vi "notes.add.vi"(8 "error in (no error)":errorcluster, 10 "midi-file-events":refnum<class "midi-file-events.lvclass">, 11 "midi-ui in":refnum<class "midi-ui.lvclass">) -> (0 "error out":errorcluster, 3 "midi-ui out":refnum<class "midi-ui.lvclass">)   [LabVIEW 2020, in "midi-ui.lvclass"]
uses:
  midi-ui.lvclass
  midi-file-events/midi-file-events.lvclass
  midi-ui.lvclass/midi-ui.ctl
  midi-file-event.midi/midi-file-event.midi.lvclass/midi-file-event.midi.ctl
  midi-file-event/midi-file-event.lvclass/midi-file-event.ctl
  midi-file-event.midi/MIDI_Messages.get.vi
  midi-file-event.midi/Data1.get.vi
  midi-file-event.midi/Data2.get.vi
  midi-file-event/uid.get.vi
  midi-file-event.midi/midi-file-event.midi.lvclass
  C:/code/LabVIEW-MIDI/lv-src/midi-file-event/midi-file-event.lvclass
  shared/midi note number.ctl
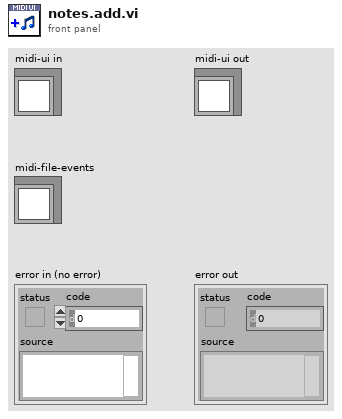
[diagram p1: front panel]
types:
  T1 = map{i32, cluster{"Note On":picture, "Note Off":picture}}
  T2 = typedef "midi-ui.lvclass/privatedata.ctl" = cluster{"White Key Length":dbl, "White Key Width":dbl, "Black Key Length":dbl, "Key Polygon Corners by Name":map{string, cluster{"x":dbl, "y":dbl}[]}, "Anticlockwise rotations [0-3] (0)":i32, "Polygon Corners by Note Name":map{T3, cluster{"x":dbl, "y":dbl}[]}, "Picture Control":refnum<vi>, "Owning VI":refnum<vi>, "Control Index":i32, "Keyboard Key Note Bounds by Note Name":map{T3, cluster{"max":dbl, "min":dbl}}, "Notes on screen":cluster{"Note":T3, "End Time":u32, "Start Time":u32}[], "Polygon Pictures by Note Name":map{T3, cluster{"Note On":picture, "Note Off":picture}}, "keyboard":picture[], "Keyboard Note Picture Index by Name":map{T3, i32}, "music":picture[], "Zoom Factor":sgl}
  T3 = typedef "midi note number.ctl" = enum8{"0 - C-1 - 8.18", "1 - C#-1 - 8.66", "2 - D-1 - 9.18", "3 - D#-1 - 9.72", "4 - E-1 - 10.30", "5 - F-1 - 10.91", "6 - F#-1 - 11.56", "7 - G-1 - 12.25", "8 - G#-1 - 12.98", "9 - A-1 - 13.75", "10 - A#-1 - 14.57", "11 - B-1 - 15.43", "12 - C0 - 16.35", "13 - C#0 - 17.32", "14 - D0 - 18.35", "15 - D#0 - 19.45", "16 - E0 - 20.60", "17 - F0 - 21.83", "18 - F#0 - 23.12", "19 - G0 - 24.50", "20 - G#0 - 25.96", "21 - A0 - 27.50", "22 - A#0 - 29.14", "23 - B0 - 30.87", "24 - C1 - 32.70", "25 - C#1 - 34.65", "26 - D1 - 36.71", "27 - D#1 - 38.89", "28 - E1 - 41.20", "29 - F1 - 43.65", "30 - F#1 - 46.25", "31 - G1 - 49.00", "32 - G#1 - 51.91", "33 - A1 - 55.00", "34 - A#1 - 58.27", "35 - B1 - 61.74", "36 - C2 - 65.41", "37 - C#2 - 69.30", "38 - D2 - 73.42", "39 - D#2 - 77.78", "40 - E2 - 82.41", "41 - F2 - 87.31", "42 - F#2 - 92.50", "43 - G2 - 98.00", "44 - G#2 - 103.83", "45 - A2 - 110.00", "46 - A#2 - 116.54", "47 - B2 - 123.47", "48 - C3 - 130.81", "49 - C#3 - 138.59", "50 - D3 - 146.83", "51 - D#3 - 155.56", "52 - E3 - 164.81", "53 - F3 - 174.61", "54 - F#3 - 185.00", "55 - G3 - 196.00", "56 - G#3 - 207.65", "57 - A3 - 220.00", "58 - A#3 - 233.08", "59 - B3 - 246.94", "60 - C4 - 261.63", "61 - C#4 - 277.18", "62 - D4 - 293.66", "63 - D#4 - 311.13", "64 - E4 - 329.63", "65 - F4 - 349.23", "66 - F#4 - 369.99", "67 - G4 - 392.00", "68 - G#4 - 415.30", "69 - A4 - 440.00", "70 - A#4 - 466.16", "71 - B4 - 493.88", "72 - C5 - 523.25", "73 - C#5 - 554.37", "74 - D5 - 587.33", "75 - D#5 - 622.25", "76 - E5 - 659.25", "77 - F5 - 698.46", "78 - F#5 - 739.99", "79 - G5 - 783.99", "80 - G#5 - 830.61", "81 - A5 - 880.00", "82 - A#5 - 932.33", "83 - B5 - 987.77", "84 - C6 - 1046.50", "85 - C#6 - 1108.73", "86 - D6 - 1174.66", "87 - D#6 - 1244.51", "88 - E6 - 1318.51", "89 - F6 - 1396.91", "90 - F#6 - 1479.98", "91 - G6 - 1567.98", "92 - G#6 - 1661.22", "93 - A6 - 1760.00", "94 - A#6 - 1864.66", "95 - B6 - 1975.53", "96 - C7 - 2093.00", "97 - C#7 - 2217.46", "98 - D7 - 2349.32", "99 - D#7 - 2489.02", "100 - E7 - 2637.02", "101 - F7 - 2793.83", "102 - F#7 - 2959.96", "103 - G7 - 3135.96", "104 - G#7 - 3322.44", "105 - A7 - 3520.00", "106 - A#7 - 3729.31", "107 - B7 - 3951.07", "108 - C8 - 4186.01", "109 - C#8 - 4434.92", "110 - D8 - 4698.63", "111 - D#8 - 4978.03", "112 - E8 - 5274.04", "113 - F8 - 5587.65", "114 - F#8 - 5919.91", "115 - G8 - 6271.93", "116 - G#8 - 6644.88", "117 - A8 - 7040.00", "118 - A#8 - 7458.62", "119 - B8 - 7902.13", "120 - C9 - 8372.02", "121 - C#9 - 8869.84", "122 - D9 - 9397.27", "123 - D#9 - 9956.06", "124 - E9 - 10548.08", "125 - F9 - 11175.30", "126 - F#9 - 11839.82", "127 - G9 - 12543.85"}
  T4 = cluster{"left":i16, "top":i16, "right":i16, "bottom":i16}
  T5 = cluster{"Note":T3, "End Time":u32, "Start Time":u32, "on uid":string, "off uid":string}
  T6 = map{T3, cluster{"Note":T3, "End Time":u32, "Start Time":u32, "on uid":string, "off uid":string}}
  T7 = map{dbl, set{refnum<class "midi-file-event.midi.lvclass">}}
  T8 = set{refnum<class "midi-file-event.midi.lvclass">}
  T9 = typedef "midi-file.lvclass/MIDI Messages.ctl" = enum8{"0(0x00)_UnassignedMidiMessage", "1(0x01)_UnassignedMidiMessage", "2(0x02)_UnassignedMidiMessage", "3(0x03)_UnassignedMidiMessage", "4(0x04)_UnassignedMidiMessage", "5(0x05)_UnassignedMidiMessage", "6(0x06)_UnassignedMidiMessage", "7(0x07)_UnassignedMidiMessage", "8(0x08)_NoteOffEvent", "9(0x09)_NoteOnEvent", "10(0x0A)_PolyphonicKeyPressure", "11(0x0B)_ControlChange", "12(0x0C)_ProgramChange", "13(0x0D)_ChannelPressure", "14(0x0E)_PitchBendChange", "15(0x0F)_SystemExclusive(SysEx)", "16(0x10)_UnassignedMidiMessage", "17(0x11)_UnassignedMidiMessage", "18(0x12)_UnassignedMidiMessage", "19(0x13)_UnassignedMidiMessage", "20(0x14)_UnassignedMidiMessage", "21(0x15)_UnassignedMidiMessage", "22(0x16)_UnassignedMidiMessage", "23(0x17)_UnassignedMidiMessage", "24(0x18)_UnassignedMidiMessage", "25(0x19)_UnassignedMidiMessage", "26(0x1A)_UnassignedMidiMessage", "27(0x1B)_UnassignedMidiMessage", "28(0x1C)_UnassignedMidiMessage", "29(0x1D)_UnassignedMidiMessage", "30(0x1E)_UnassignedMidiMessage", "31(0x1F)_UnassignedMidiMessage", "32(0x20)_UnassignedMidiMessage", "33(0x21)_UnassignedMidiMessage", "34(0x22)_UnassignedMidiMessage", "35(0x23)_UnassignedMidiMessage", "36(0x24)_UnassignedMidiMessage", "37(0x25)_UnassignedMidiMessage", "38(0x26)_UnassignedMidiMessage", "39(0x27)_UnassignedMidiMessage", "40(0x28)_UnassignedMidiMessage", "41(0x29)_UnassignedMidiMessage", "42(0x2A)_UnassignedMidiMessage", "43(0x2B)_UnassignedMidiMessage", "44(0x2C)_UnassignedMidiMessage", "45(0x2D)_UnassignedMidiMessage", "46(0x2E)_UnassignedMidiMessage", "47(0x2F)_UnassignedMidiMessage", "48(0x30)_UnassignedMidiMessage", "49(0x31)_UnassignedMidiMessage", "50(0x32)_UnassignedMidiMessage", "51(0x33)_UnassignedMidiMessage", "52(0x34)_UnassignedMidiMessage", "53(0x35)_UnassignedMidiMessage", "54(0x36)_UnassignedMidiMessage", "55(0x37)_UnassignedMidiMessage", "56(0x38)_UnassignedMidiMessage", "57(0x39)_UnassignedMidiMessage", "58(0x3A)_UnassignedMidiMessage", "59(0x3B)_UnassignedMidiMessage", "60(0x3C)_UnassignedMidiMessage", "61(0x3D)_UnassignedMidiMessage", "62(0x3E)_UnassignedMidiMessage", "63(0x3F)_UnassignedMidiMessage", "64(0x40)_UnassignedMidiMessage", "65(0x41)_UnassignedMidiMessage", "66(0x42)_UnassignedMidiMessage", "67(0x43)_UnassignedMidiMessage", "68(0x44)_UnassignedMidiMessage", "69(0x45)_UnassignedMidiMessage", "70(0x46)_UnassignedMidiMessage", "71(0x47)_UnassignedMidiMessage", "72(0x48)_UnassignedMidiMessage", "73(0x49)_UnassignedMidiMessage", "74(0x4A)_UnassignedMidiMessage", "75(0x4B)_UnassignedMidiMessage", "76(0x4C)_UnassignedMidiMessage", "77(0x4D)_UnassignedMidiMessage", "78(0x4E)_UnassignedMidiMessage", "79(0x4F)_UnassignedMidiMessage", "80(0x50)_UnassignedMidiMessage", "81(0x51)_UnassignedMidiMessage", "82(0x52)_UnassignedMidiMessage", "83(0x53)_UnassignedMidiMessage", "84(0x54)_UnassignedMidiMessage", "85(0x55)_UnassignedMidiMessage", "86(0x56)_UnassignedMidiMessage", "87(0x57)_UnassignedMidiMessage", "88(0x58)_UnassignedMidiMessage", "89(0x59)_UnassignedMidiMessage", "90(0x5A)_UnassignedMidiMessage", "91(0x5B)_UnassignedMidiMessage", "92(0x5C)_UnassignedMidiMessage", "93(0x5D)_UnassignedMidiMessage", "94(0x5E)_UnassignedMidiMessage", "95(0x5F)_UnassignedMidiMessage", "96(0x60)_UnassignedMidiMessage", "97(0x61)_UnassignedMidiMessage", "98(0x62)_UnassignedMidiMessage", "99(0x63)_UnassignedMidiMessage", "100(0x64)_UnassignedMidiMessage", "101(0x65)_UnassignedMidiMessage", "102(0x66)_UnassignedMidiMessage", "103(0x67)_UnassignedMidiMessage", "104(0x68)_UnassignedMidiMessage", "105(0x69)_UnassignedMidiMessage", "106(0x6A)_UnassignedMidiMessage", "107(0x6B)_UnassignedMidiMessage", "108(0x6C)_UnassignedMidiMessage", "109(0x6D)_UnassignedMidiMessage", "110(0x6E)_UnassignedMidiMessage", "111(0x6F)_UnassignedMidiMessage", "112(0x70)_UnassignedMidiMessage", "113(0x71)_UnassignedMidiMessage", "114(0x72)_UnassignedMidiMessage", "115(0x73)_UnassignedMidiMessage", "116(0x74)_UnassignedMidiMessage", "117(0x75)_UnassignedMidiMessage", "118(0x76)_UnassignedMidiMessage", "119(0x77)_UnassignedMidiMessage", "120(0x78)_UnassignedMidiMessage", "121(0x79)_UnassignedMidiMessage", "122(0x7A)_UnassignedMidiMessage", "123(0x7B)_UnassignedMidiMessage", "124(0x7C)_UnassignedMidiMessage", "125(0x7D)_UnassignedMidiMessage", "126(0x7E)_UnassignedMidiMessage", "127(0x7F)_UnassignedMidiMessage"}
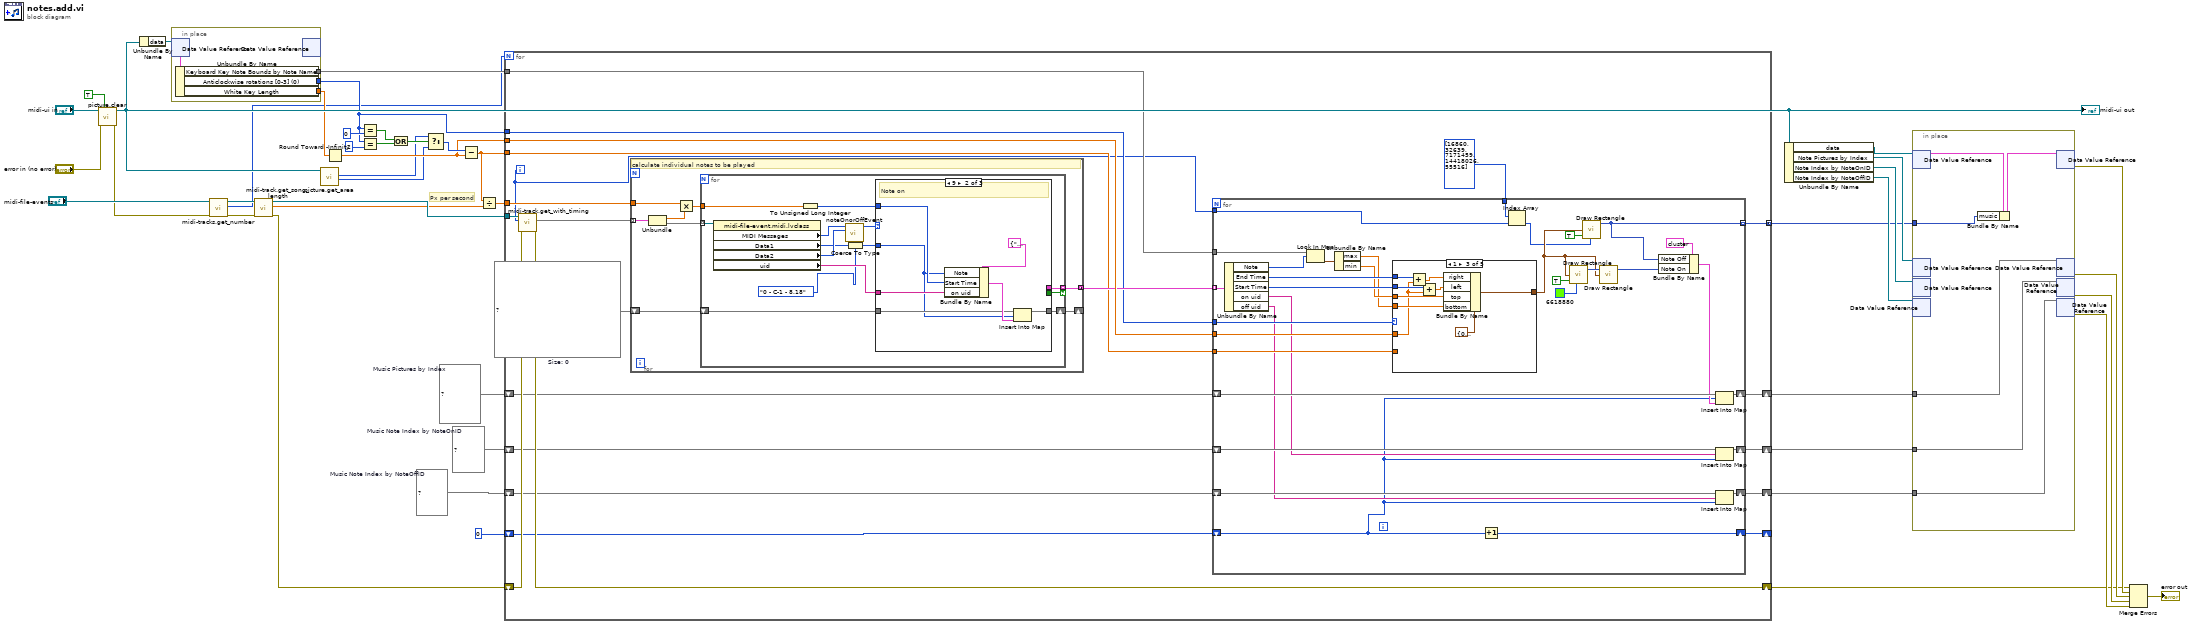
[diagram p0: block diagram]
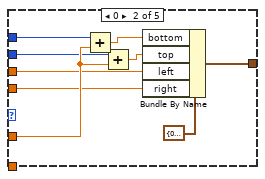
[diagram p3: hidden frame]
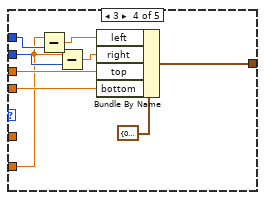
[diagram p4: hidden frame]
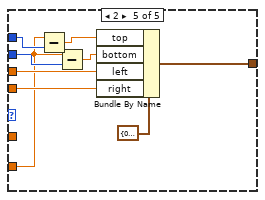
[diagram p5: hidden frame]
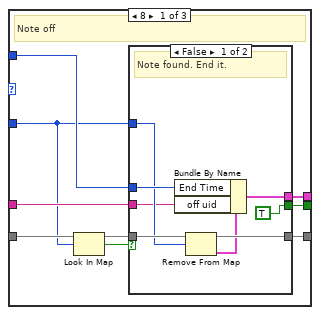
[diagram p6: hidden frame]
diagram:
  w7 = map{string, i32} {}  # Music Note Index by NoteOffID
  w9 = T1 {}  # Music Pictures by Index
  w8 = map{string, i32} {}  # Music Note Index by NoteOnID
  # "Px per second"
  n1 = call "picture.clear.vi"("Keep Keyboard? (T)"=TRUE, "error in"="error in (no error)", "midi-ui in"="midi-ui in") -> ("error out"=w14:errorcluster, "midi-ui out"=w32:refnum<class "midi-ui.lvclass">)  [unwired: 7 in]
  "midi-ui out" <- w32
  n2 = Unbundle By Name(w32) -> ("data"=w31:refnum<data-value>)
  n3 = in-place {
    in-place-border: [w48] -> w30
    in-place-border: [w47] -> w29
    in-place-border: [w46] -> w28
    n4 = in-place-dvr #1(w31) -> (w49:T2)  [unwired: 1 out]
    n5 = Unbundle By Name(w49) -> ("Keyboard Key Note Bounds by Note Name"=w46:map{T3, cluster{"max":dbl, "min":dbl}}, "Anticlockwise rotations [0-3] (0)"=w48:i32, "White Key Length"=w47:dbl)
    n6 = in-place-dvr #1() -> ()  [unwired: 1 in, 2 out]
  }
  n7 = call "midi-tracks.get_number.vi"("error in (no error)"=w14, "midi-file-events in"="midi-file-events") -> ("error out"=w17:errorcluster, "Numer of Tracks"=w10:i32, "midi-file-events out"=w18:refnum<class "midi-file-events.lvclass">)  [unwired: 7 in]
  n8 = call "midi-track.get_song_length.vi"("error in (no error)"=w17, "midi-file-events in"=w18) -> ("error out"=w16:errorcluster, "Song Length (s)"=w11:dbl, "midi-file-events out"=w15:refnum<class "midi-file-events.lvclass">)  [unwired: 7 in]
  n9 = call "picture.get_area.vi"("midi-ui in"=w32) -> ("Bounds:Area Width"=w33:u32, "Bounds:Area Height"=w34:u32)  [unwired: 7 in, 2 out]
  n10 = Round Toward -Infinity(1:w29) -> (0:w38:dbl)
  n11 = Equal?(x=w30, y=0) -> (x = y?=w43:bool)
  n12 = Equal?(x=w30, y=2) -> (x = y?=w42:bool)
  n13 = Or(x=w43, y=w42) -> (x .or. y?=w41:bool)
  n14 = Select(t=w34, s=w41, f=w33) -> (s? t:f=w40:u32)
  n15 = Subtract(x=w40, y=w38) -> (x-y=w12:dbl)
  n16 = Divide(x=w12, y=w11) -> (x/y=w39:dbl)
  n17 = for {
    N: w10 -> [_]
    tunnel: w39 -> [w71]
    tunnel: w38 -> [w69]
    tunnel: w30 -> [w67]
    tunnel: w28 -> [w66]
    tunnel: w15 -> [w63]
    tunnel: w12 -> [w61]
    shift-right: [w62] -> w13
    shift-left: w16 -> [w64]
    shift-right: [w55] -> w4
    shift-left: w9 -> [w60]
    shift-right: [w57] -> w6
    shift-left: w8 -> [w59]
    shift-right: [w56] -> w5
    shift-left: w7 -> [w58]
    tunnel: [w54] -> w3 mode=concatenating
    shift-right: [w52] -> _
    shift-left: 0 -> [w53]
    i -> [w50]
    w70 = T6 {}  # Size: 0
    n18 = call "midi-track.get_with_timing.vi"("error in (no error)"=w64, "Track Number"=w50, "midi-file-events in"=w63) -> ("error out"=w62:errorcluster, "Events by time"=w65:T7)  [unwired: 6 in, 1 out]
    n19 = for {
      tunnel: w65 -> [w144] mode=indexing
      shift-right: [w147] -> _
      shift-left: w70 -> [w148]
      tunnel: [w146] -> w68 mode=concatenating
      tunnel: w71 -> [w145]
      # "calculate individual notes to be played"
      n20 = Unbundle(w144) -> ("Timestamp"=w143:dbl, w142:T8)
      n21 = Multiply(x=w145, y=w143) -> (x*y=w141:dbl)
      n22 = for {
        tunnel: w141 -> [w160]
        tunnel: [w159] -> w146 mode=indexing if=w152
        tunnel: w142 -> [w153] mode=indexing
        shift-right: [w161] -> w147
        shift-left: w148 -> [w162]
        n23 = property class="midi-file-event.midi.lvclass"(reference=w153) -> ("MIDI Messages"=w156:T9, "Data1"=w151:u8, "Data2"=w155:u8, "uid"=w154:string)  [unwired: 1 in, 2 out]
        n24 = To Unsigned Long Integer(number=w160) -> (unsigned 32bit integer=w157:u32)
        n25 = call "noteOnorOffEvent.vi"("Volume"=w155, "MIDI Message"=w156) -> ("Midi Message"=w158:u16)  [unwired: 9 in]
        n26 = Coerce To Type(0:w151, 1:midi_note_number."0 - C-1 - 8.18" ("Note")) -> (2:w150:T3)
        n27 = case shown="9" w158 {
          tunnel: w162 -> [w166 w182 w187]
          tunnel: [w170 w185 w187] -> w161
          tunnel: w150 -> [w163 w181 _]
          tunnel: w157 -> [w169 w186 _]
          tunnel: [w168 _ _] -> w159
          tunnel: [w167 _ _] -> w152
          tunnel: w154 -> [w164 w183 _]
          frame 8 {
            # "Note off"
            n28 = Look In Map(map=w166, key=w163) -> (key not found?=w165:bool)  [unwired: 1 in, 1 out]
            n29 = case shown="False" w165 {
              tunnel: [w174 w179] -> w170
              tunnel: w166 -> [w175 w179]
              tunnel: w169 -> [w178 _]
              tunnel: [w177 _] -> w168
              tunnel: [TRUE _] -> w167
              tunnel: w163 -> [w173 _]
              tunnel: w164 -> [w171 _]
              frame False {
                # "Note found. End it."
                n30 = Remove From Map(10:w173, 11:w175) -> (1:w172:T5, 3:w174:T6)  [unwired: 1 out]
                n31 = Bundle By Name(cluster=w172, "End Time"=w178, "off uid"=w171) -> (w177:T5)
              }
              frame True {
                # "Not found so ignore"
              }
            }
          }
          frame 9 {
            # "Note on"
            n32 = Bundle By Name(cluster=T5 {"Note"=enum."0 - C-1 - 8.18", "End Time"=0, "Start Time"=0, "on uid"="", "off uid"=""}, "Note"=w181, "Start Time"=w186, "on uid"=w183) -> (w184:T5)
            n33 = Insert Into Map(map in=w182, key=w181, value=w184) -> (map out=w185:T6)  [unwired: 2 out]
          }
          frame Default {
          }
        }
      }
    }
    n34 = for {
      tunnel: w68 -> [w104] mode=indexing
      tunnel: w66 -> [w80]
      tunnel: w67 -> [w98]
      tunnel: w69 -> [w97]
      tunnel: w61 -> [w96]
      shift-right: [w93] -> w55
      shift-left: w60 -> [w94]
      shift-right: [w92] -> w57
      shift-left: w59 -> [w95]
      shift-right: [w82] -> w56
      shift-left: w58 -> [w83]
      tunnel: [w78] -> w54 mode=indexing
      shift-right: [w77] -> w52
      shift-left: w53 -> [w76]
      tunnel: u32[] [16860, 32639, 7171459, 14418026, 55516] ("color(black)") -> [w75]
      tunnel: w50 -> [w73]
      n35 = Unbundle By Name(w104) -> ("Note"=w72:T3, "End Time"=w102:u32, "Start Time"=w103:u32, "on uid"=w84:string, "off uid"=w81:string)
      n36 = Look In Map(map=w80, key=w72) -> (value=w101:cluster{"max":dbl, "min":dbl})  [unwired: 1 in, 1 out]
      n37 = Unbundle By Name(w101) -> ("max"=w99:dbl, "min"=w100:dbl)
      n38 = case shown="1" w98 {
        tunnel: w103 -> [_ w108 w117 w126 w135]
        tunnel: w102 -> [_ w110 w118 w127 w136]
        tunnel: [_ w105 w121 w130 w139] -> w87
        tunnel: w100 -> [_ w107 w120 w129 w138]
        tunnel: w99 -> [_ w106 w119 w128 w137]
        tunnel: w97 -> [_ w109 w114 _ _]
        tunnel: w96 -> [_ _ _ w123 w132]
        frame Default {
        }
        frame 0 {
          n39 = Add(x=w110, y=w109) -> (x+y=w112:dbl)
          n40 = Add(x=w108, y=w109) -> (x+y=w111:dbl)
          n41 = Bundle By Name(cluster=T4 {"left"=0, "top"=0, "right"=0, "bottom"=0} ("rect"), "bottom"=w112, "top"=w111, "left"=w107, "right"=w106) -> (w105:T4)
        }
        frame 1 {
          n42 = Add(x=w118, y=w114) -> (x+y=w116:dbl)
          n43 = Add(x=w117, y=w114) -> (x+y=w115:dbl)
          n44 = Bundle By Name(cluster=T4 {"left"=0, "top"=0, "right"=0, "bottom"=0} ("rect"), "right"=w116, "left"=w115, "top"=w120, "bottom"=w119) -> (w121:T4)
        }
        frame 3 {
          n45 = Subtract(x=w123, y=w127) -> (x-y=w125:dbl)
          n46 = Subtract(x=w123, y=w126) -> (x-y=w124:dbl)
          n47 = Bundle By Name(cluster=T4 {"left"=0, "top"=0, "right"=0, "bottom"=0} ("rect"), "left"=w125, "right"=w124, "top"=w129, "bottom"=w128) -> (w130:T4)
        }
        frame 2 {
          n48 = Subtract(x=w132, y=w136) -> (x-y=w134:dbl)
          n49 = Subtract(x=w132, y=w135) -> (x-y=w133:dbl)
          n50 = Bundle By Name(cluster=T4 {"left"=0, "top"=0, "right"=0, "bottom"=0} ("rect"), "top"=w134, "bottom"=w133, "left"=w138, "right"=w137) -> (w139:T4)
        }
      }
      n51 = Increment(x=w76) -> (x+1=w77:i32)
      n52 = Index Array(array=w75, index=w73) -> (element=w74:u32)
      n53 = call <vilib>:"Draw Rectangle.vi"("rect"=w87, "fill?(F)"=TRUE, "color(black)"=u32 6618880) -> ("new picture"=w88:picture)  [unwired: 6 in]
      n54 = call <vilib>:"Draw Rectangle.vi"("rect"=w87, "fill?(F)"=TRUE, "color(black)"=w74) -> ("new picture"=w78:picture)  [unwired: 6 in]
      n55 = call <vilib>:"Draw Rectangle.vi"("picture"=w88, "rect"=w87) -> ("new picture"=w86:picture)  [unwired: 7 in]
      n56 = Bundle By Name(cluster=cluster{"Note On":picture, "Note Off":picture} {"Note On"=bytes[0], "Note Off"=bytes[0]} ("value"), "Note Off"=w78, "Note On"=w86) -> (w85:cluster{"Note On":picture, "Note Off":picture})
      n57 = Insert Into Map(map in=w94, key=w76, value=w85) -> (map out=w93:T1)  [unwired: 2 out]
      n58 = Insert Into Map(map in=w95, key=w84, value=w76) -> (map out=w92:map{string, i32})  [unwired: 2 out]
      n59 = Insert Into Map(map in=w83, key=w81, value=w76) -> (map out=w82:map{string, i32})  [unwired: 2 out]
    }
  }
  n60 = Unbundle By Name(w32) -> ("data"=w35:refnum<data-value>, "Note Pictures by Index"=w27:refnum<data-value>, "Note Index by NoteOnID"=w26:refnum<data-value>, "Note Index by NoteOffID"=w25:refnum<data-value>)
  n61 = in-place {
    in-place-border: w5 -> [w191]
    in-place-border: w6 -> [w190]
    in-place-border: w4 -> [w189]
    in-place-border: w3 -> [w188]
    n62 = in-place-dvr #2(w35) -> (w193:T2)  [unwired: 1 out]
    n63 = in-place-dvr #3(w27) -> ()  [unwired: 2 out]
    n64 = in-place-dvr #4(w26) -> ()  [unwired: 2 out]
    n65 = in-place-dvr #5(w25) -> ()  [unwired: 2 out]
    n66 = Bundle By Name(cluster=w193, "music"=w188) -> (w192:T2)
    n67 = in-place-dvr #2(w192) -> (w24:errorcluster)  [unwired: 1 out]
    n68 = in-place-dvr #3(w189) -> (w23:errorcluster)  [unwired: 1 out]
    n69 = in-place-dvr #4(w190) -> (w22:errorcluster)  [unwired: 1 out]
    n70 = in-place-dvr #5(w191) -> (w21:errorcluster)  [unwired: 1 out]
  }
  n71 = Merge Errors(w13, w24, w23, w22, w21) -> (→"error out":errorcluster)
